vi "Find Parent Struct.vi"(8 "error in (no error)":errorcluster, 11 "Objects in":T1[](array[typedef])) -> (0 "error out":errorcluster, 3 "Found Parent Struct":T1[](array[typedef]))   [LabVIEW 2023, in "VIDoc Parsing.lvlib" / "Structure Reporter.lvlib"]
uses:
  Structure Reporter.lvlib
  Structure Result 2.ctl
panel:
  in  "Tab Control":enum32{"Array in", "Parent Structs Found"}(tab)
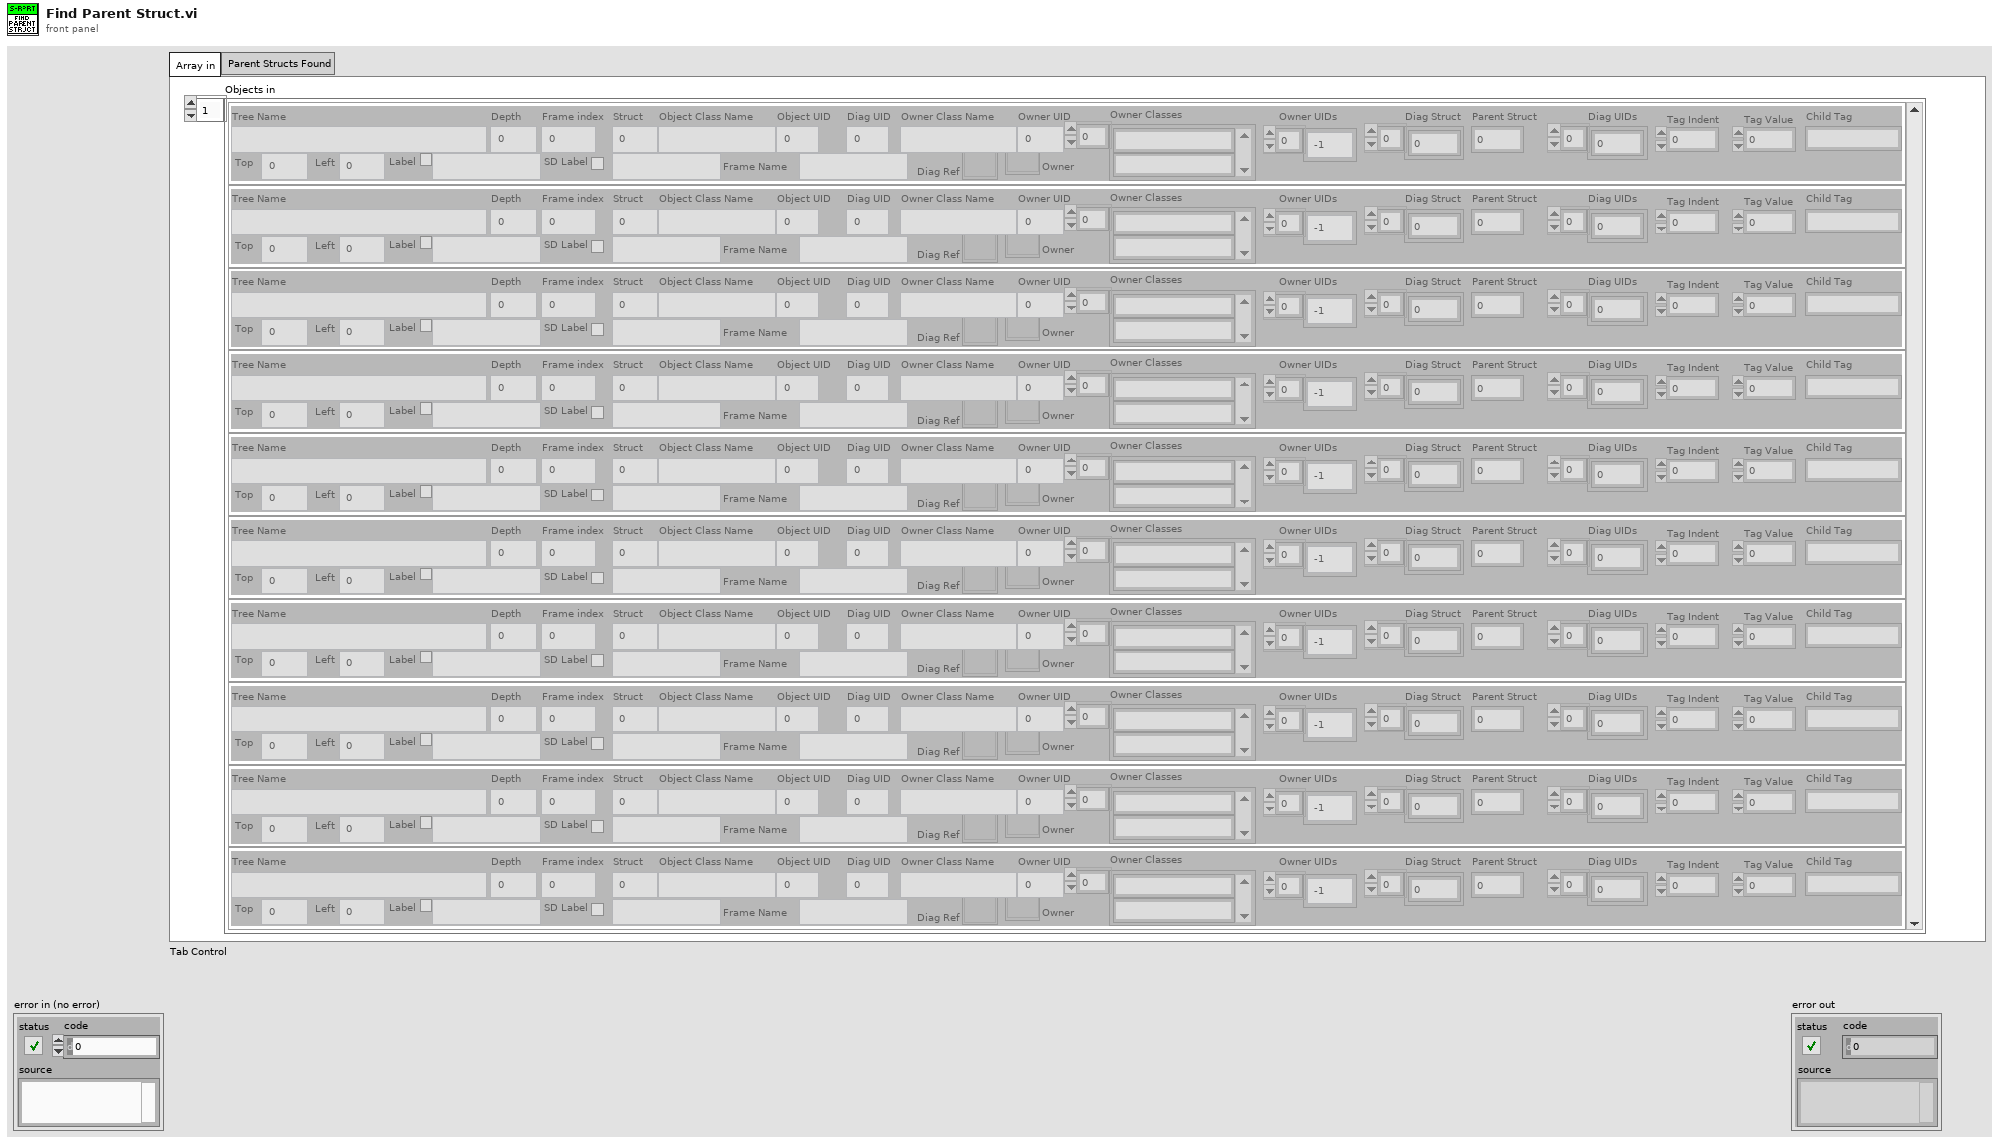
[diagram p1: front panel]
types:
  T1 = typedef "VIDoc Parsing.lvlib/Structure Reporter.lvlib/Structure Result 2.ctl" = cluster{"Depth":i32, "Top":i32, "Left":i32, "Frame index":i32, "Struct":i32, "Object Class Name":string, "Object UID":i32, "Label Visible":bool, "Object Label":string, "SD Label Visible":bool, "Object SD Label":string, "Frame Name":string, "Diag UID":i32, "Owner Class Name":string, "Owner UID":i32, "Diag Struct":i32[], "Parent Struct":i32, "Diag UIDs":i32[], "Tree Name":string, "Diag Ref":refnum<vi>, "Owner Classes":string[], "Owner":refnum<vi>, "Owner UIDs":i32[], "Tag Indent":i32, "Tag Value":i32, "Child Tag":string}
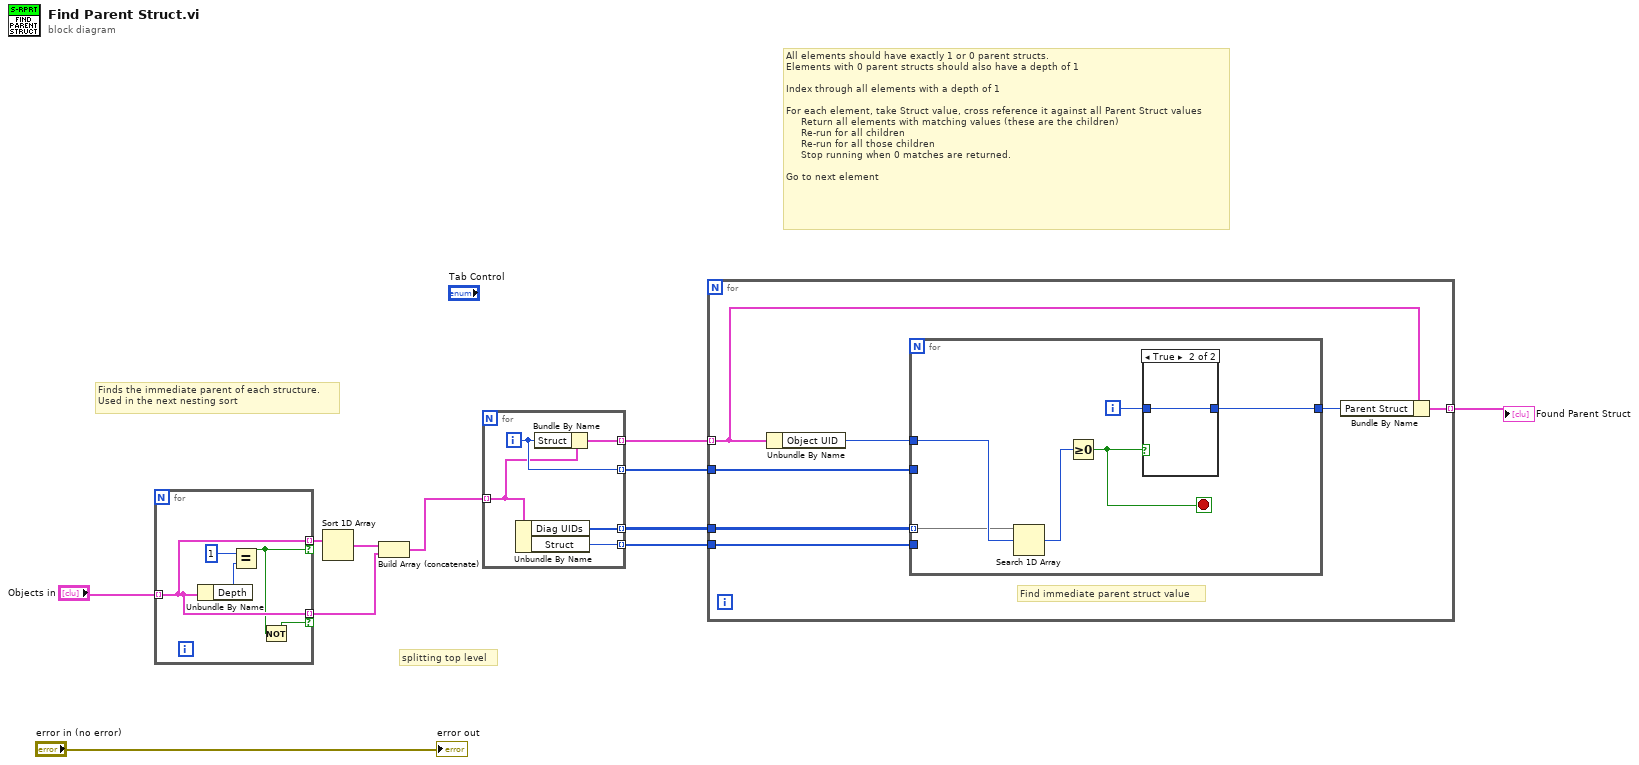
[diagram p0: block diagram]
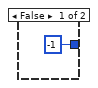
[diagram p2: hidden frame]
diagram:
  # "Finds the immediate parent of each structure.\nUsed in the next nesting sort"
  # "All elements should have exactly 1 or 0 parent structs.\nElements with 0 parent structs should also have a depth of 1 \n\nIndex through all elements with a depth of 1\n\nFor each element, take Struct value, cross reference it against all Parent Struct values\n     Return all elements with matching values (these are the children)\n     Re-run for all children\n     Re-run for all those children\n     Stop running when 0 matches are returned.\n\nGo to next element"
  # "splitting top level"
  n1 = for {
    tunnel: "Objects in" -> [w14] mode=indexing
    tunnel: [w14] -> w10 mode=indexing if=w13
    tunnel: [w14] -> w7 mode=indexing if=w12
    n2 = Unbundle By Name(w14) -> ("Depth"=w16:i32)
    n3 = Equal?(x=1, y=w16) -> (x = y?=w13:bool)
    n4 = Not(x=w13) -> (.not. x?=w12:bool)
  }
  n5 = Sort 1D Array(array=w10) -> (sorted array=w8:T1[])
  n6 = Build Array (concatenate)(w8, w7) -> (w6:T1[])
  n7 = for {
    tunnel: w6 -> [w20] mode=indexing
    tunnel: [w21] -> w11 mode=indexing
    tunnel: [w19] -> w5 mode=indexing
    tunnel: [w18] -> w4 mode=indexing
    tunnel: [w17] -> w3 mode=indexing
    i -> [w21]
    n8 = Unbundle By Name(w20) -> ("Diag UIDs"=w18:i32[], "Struct"=w17:i32)
    n9 = Bundle By Name(cluster=w20, "Struct"=w21) -> (w19:T1)
  }
  n10 = for {
    tunnel: w5 -> [w28] mode=indexing
    tunnel: w4 -> [w26]
    tunnel: [w27] -> w1 mode=indexing
    tunnel: w11 -> [w24]
    tunnel: w3 -> [w23]
    # "Find immediate parent struct value"
    n11 = Unbundle By Name(w28) -> ("Object UID"=w25:i32)
    n12 = for {
      tunnel: w25 -> [w34]
      tunnel: w26 -> [w33] mode=indexing
      tunnel: w24 -> [_]
      tunnel: w23 -> [_]
      tunnel: [w30] -> w22
      i -> [w32]
      stop <- w29 stop-if-true
      n13 = Search 1D Array(1D array=w33, element=w34) -> (index of element=w31:i32)  [unwired: 1 in]
      n14 = Greater Or Equal To 0?(x=w31) -> (x >= 0?=w29:bool)
      n15 = case shown="True" w29 {
        tunnel: [-1 w36] -> w30
        tunnel: w32 -> [_ w36]
        frame False {
        }
        frame True {
        }
      }
    }
    n16 = Bundle By Name(cluster=w28, "Parent Struct"=w22) -> (w27:T1)
  }
  "Found Parent Struct" <- w1
  "error out" <- "error in (no error)"
